vi "json_is_empty.vi"(1 "variant in":variant) -> (0 "is_empty?":bool)   [LabVIEW 2017, in "rethinkdb.lvlib"]
uses:
  rethinkdb.lvlib
  <vilib>/Utility/Data Type/NI_Data Type.lvlib
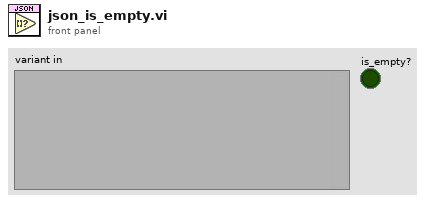
[diagram p1: front panel]
types:
  T1 = typedef "NI_Data Type.lvlib/Data Type.ctl" = enum8{"Invalid Type", "Void", "I8", "I16", "I32", "I64", "U8", "U16", "U32", "U64", "Single Float", "Double Float", "Extended Float", "Single Complex", "Double Complex", "Extended Complex", "Enum U8", "Enum U16", "Enum U32", "Enum U64", "Single Float With Unit", "Double Float With Unit", "Extended Float With Unit", "Single Complex with Unit", "Double Complex with Unit", "Extended Complex with Unit", "Boolean", "String", "Path", "Picture", "Tag", "Array", "Cluster", "Variant", "LV Variant", "Waveform", "Timestamp", "Digital Waveform", "Digital Data", "ExpressData", "Refnum", "External Data", "VI", "Poly VI", "LabVIEW Class Instance", "Fixed Point"}
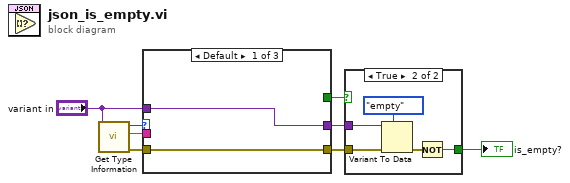
[diagram p0: block diagram]
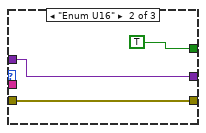
[diagram p2: hidden frame]
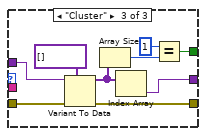
[diagram p3: hidden frame]
diagram:
  n1 = call <vilib>:"Get Type Information.vi"("Variant"="variant in") -> ("error out"=w7:errorcluster, "Name"=w5:string, "Type"=w6:T1)  [unwired: 6 in, 2 out]
  n2 = case shown="Default" w6 {
    tunnel: w7 -> [w9 w13 w22]
    tunnel: "variant in" -> [w10 w12 w21]
    tunnel: w5 -> [_ _ _]
    tunnel: [w9 w13 w19] -> w3
    tunnel: [w10 w12 w15] -> w2
    tunnel: [_ TRUE w14] -> w1
    frame Default {
    }
    frame "Enum U16" {
    }
    frame "Cluster" {
      n3 = Variant To Data(error in=w22, type=variant[] [], Variant=w21) -> (data=w16:variant[], error out=w19:errorcluster)
      n4 = Array Size(array=w16) -> (size(s)=w18:i32)
      n5 = Index Array(array=w16) -> (element=w15:variant)  [unwired: 1 in]
      n6 = Equal?(x=1 ("y"), y=w18) -> (x = y?=w14:bool)
    }
  }
  n7 = case shown="True" w1 {
    tunnel: [_ w27] -> w4
    tunnel: w3 -> [_ w25]
    tunnel: w2 -> [_ w24]
    frame False {
    }
    frame True {
      n8 = Variant To Data(error in=w25, type=enum16{"empty"}."empty", Variant=w24) -> (error out=w26:errorcluster)  [unwired: 1 out]
      n9 = Not(x=w26) -> (.not. x?=w27:bool)
    }
  }
  "is_empty?" <- w4
